vi "ConvertePacoteCRIO.vi"(0 "DadosCanais":T1[](array[typedef]), 2 "Sinais":waveform(dbl)[](array[waveform]), 4 "Tx Aquisicao":dbl, 5 "numBloco":i32) -> (16 "Tipo_PacoteModuloCRIO":T3)   [LabVIEW 2017]
uses:
  Typedefs/Tipo_PacoteModuloCRIO.ctl
  Typedefs/Tipo_moduloCRIO.ctl
  Typedefs/Tipo_DadosCanal.ctl
  Typedefs/Tipo_TipoSinalSimulado.ctl
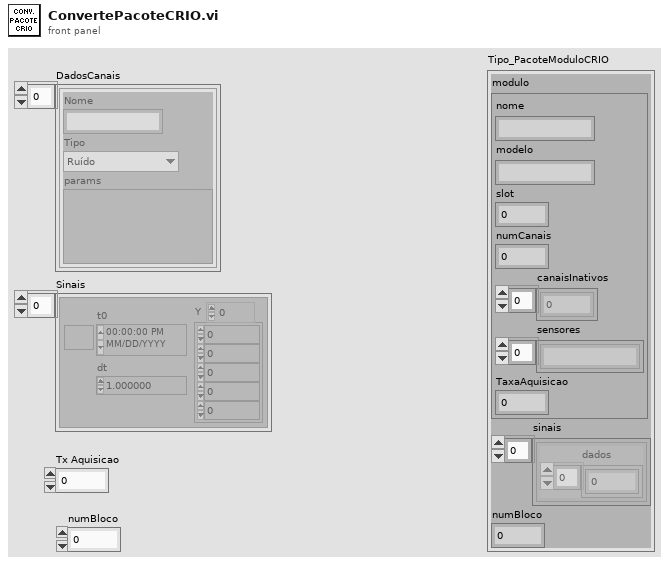
[diagram p1: front panel]
types:
  T1 = typedef "Tipo_DadosCanal.ctl" = cluster{"Nome":string, "Tipo":T2, "params":variant}
  T2 = typedef "Tipo_TipoSinalSimulado.ctl" = enum16{"Ruído", "Fasor", "Senóide", "Composto", "AM", "Proximidade", "Entreferro"}
  T3 = typedef "Tipo_PacoteModuloCRIO.ctl" = cluster{"modulo":T4, "sinais":cluster{"dados":sgl[]}[], "numBloco":i32}
  T4 = typedef "Tipo_moduloCRIO.ctl" = cluster{"nome":string, "modelo":string, "slot":i32, "numCanais":i32, "canaisInativos":i32[], "sensores":string[], "TaxaAquisicao":dbl}
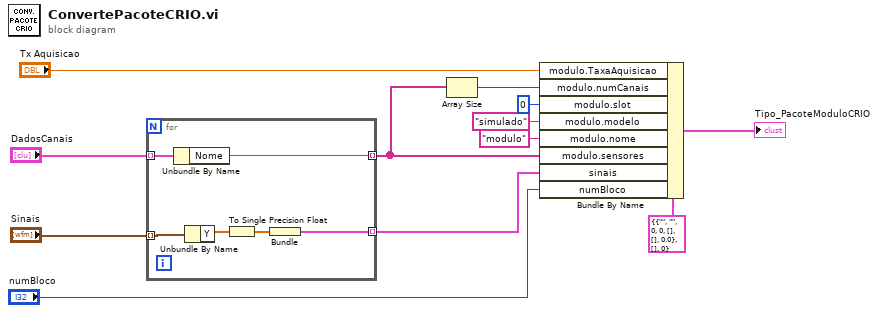
[diagram p0: block diagram]
diagram:
  n1 = for {
    tunnel: "DadosCanais" -> [w14] mode=indexing
    tunnel: "Sinais" -> [w18] mode=indexing
    tunnel: [w16] -> w8 mode=indexing
    tunnel: [w13] -> w4 mode=indexing
    n2 = Unbundle By Name(w14) -> ("Nome"=w13:string)
    n3 = Unbundle By Name(w18) -> ("Y"=w17:dbl[])
    n4 = To Single Precision Float(number=w17) -> (single precision float=w15:sgl[])
    n5 = Bundle(w15) -> (w16:cluster{sgl[]})  [unwired: 1 in]
  }
  n6 = Array Size(array=w4) -> (size(s)=w3:i32)
  n7 = Bundle By Name(cluster=T3 {"modulo"={"nome"="", "modelo"="", "slot"=0, "numCanais"=0, "canaisInativos"=[], "sensores"=[], "TaxaAquisicao"=0.0}, "sinais"=[], "numBloco"=0} ("Tipo_PacoteModuloCRIO"), "modulo.TaxaAquisicao"="Tx Aquisicao", "modulo.numCanais"=w3, "modulo.slot"=0, "modulo.modelo"="simulado", "modulo.nome"="modulo", "modulo.sensores"=w4, "sinais"=w8, "numBloco"="numBloco") -> (→"Tipo_PacoteModuloCRIO":T3)
